vi "Set Segmented Log Type.vi"(8 "error in (no error)":errorcluster, 10 "Segmented Log Type":T1, 11 "Segmented Log in":refnum<class "Segmented Log.lvclass">) -> (0 "error out":errorcluster, 3 "Segmented Log out":refnum<class "Segmented Log.lvclass">)   [LabVIEW 2012, in "Waveform Data Logger Engine.lvlib" / "Segmented Log.lvclass"]
uses:
  Segmented Log.lvclass
  Segmented Log Type.ctl
  Segmented Log.lvclass/Segmented Log.ctl
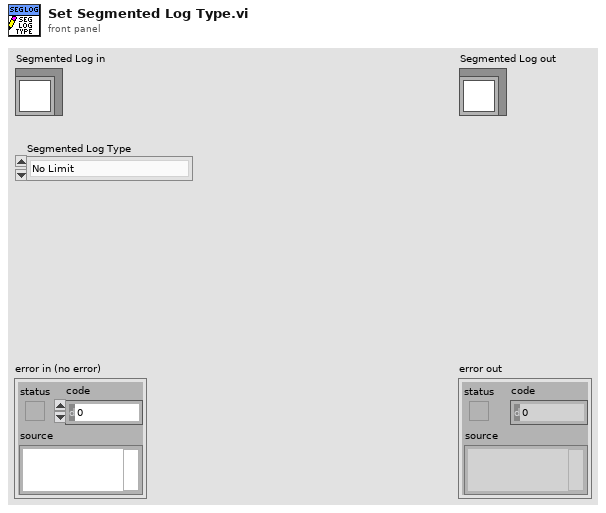
[diagram p1: front panel]
types:
  T1 = typedef "Waveform Data Logger Engine.lvlib/Segmented Log.lvclass/Segmented Log Type.ctl" = enum16{"No Limit", "Footprint", "Time"}
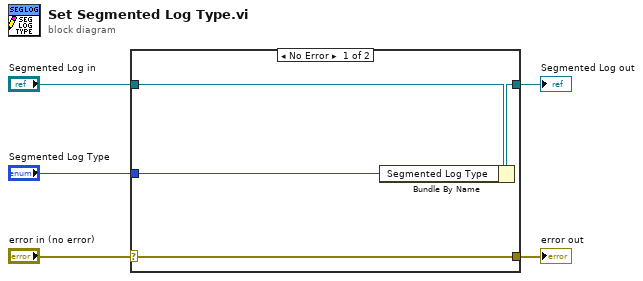
[diagram p0: block diagram]
diagram:
  n1 = case shown="No Error" "error in (no error)" {
    selector: "error in (no error)" -> [w9 w10]
    tunnel: [w9 w10] -> w4
    tunnel: [w7 w11] -> w2
    tunnel: "Segmented Log in" -> [w8 w11]
    tunnel: "Segmented Log Type" -> [w6 _]
    frame No Error {
      n2 = Bundle By Name(cluster=w8, "Segmented Log Type"=w6) -> (w7:refnum<class "Segmented Log.lvclass">)
    }
    frame Error {
    }
  }
  "error out" <- w4
  "Segmented Log out" <- w2
